vi "test_output_format.vi"() -> ()   [LabVIEW 2025]
panel:
  out "I":fxp<+/-,18,1>
  in  "Data in":fxp<+/-,32,14>[](array[numeric])=[0.0, 0.0]
  in  "factor":u16
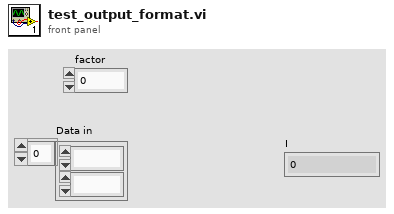
[diagram p1: front panel]
types:
  T1 = typedef "IQ-1element.ctl" = T2[]
  T2 = typedef "niInstr DSP v1 Shared.lvlib/IQ Data.ctl" = cluster{"I":fxp<+/-,18,1>, "Q":fxp<+/-,18,1>, "overflow":bool}
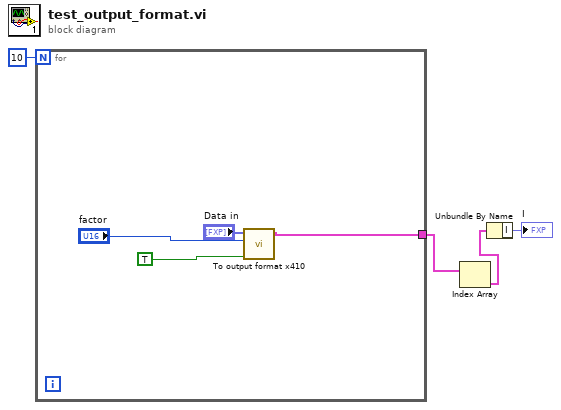
[diagram p0: block diagram]
diagram:
  n1 = for {
    N: 10 -> [_]
    tunnel: [w8] -> w3
    n2 = call "To output format x410.vi"("input valid"=TRUE ("valid in"), "factor"="factor", "Data in"="Data in") -> ("Data out"=w8:T1)  [unwired: 7 in, 1 out]
  }
  n3 = Index Array(array=w3) -> (element=w2:T2)  [unwired: 1 in]
  n4 = Unbundle By Name(w2) -> ("I"=→"I":fxp<+/-,18,1>)
